vi "小数字符串变整数字符串.vi"(11 "字符串":string) -> (3 "十进制整型字符串":string)   [LabVIEW 2017]
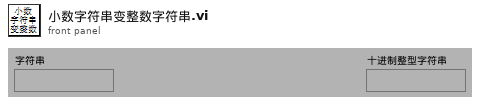
[diagram p1: front panel]
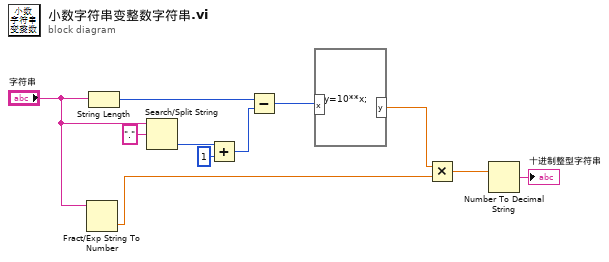
[diagram p0: block diagram]
diagram:
  n1 = Fract/Exp String To Number(string="字符串") -> (number=w3:dbl)  [unwired: 3 in, 1 out]
  n2 = String Length(string="字符串") -> (length=w11:i32)
  n3 = Search/Split String(string="字符串", search string/char (-)="." ("正则表达式")) -> (offset of match=w8:i32)  [unwired: 1 in, 2 out]
  n4 = Add(x=w8, y=1) -> (x+y=w6:i32)
  n5 = Subtract(x=w11, y=w6) -> (x-y=w5:i32)
  n6 = formula code="y=10**x;"("x"=w5) -> ("y"=w4:dbl)
  n7 = Multiply(x=w4, y=w3) -> (x*y=w2:dbl)
  n8 = Number To Decimal String(number=w2) -> (decimal integer string=→"十进制整型字符串":string)  [unwired: 1 in]
